vi "global.vi"() -> ()   [LabVIEW 2015]
panel:
  out "stop":bool
  out "crashed":bool
  out "FG Data":T1
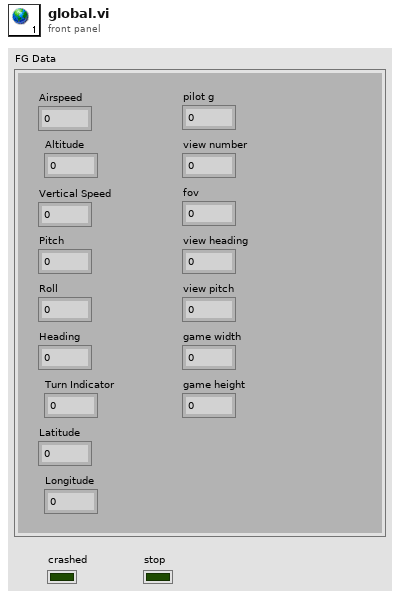
[diagram p1: front panel]
types:
  T1 = cluster{"Airspeed":dbl, "Altitude":dbl, "Vertical Speed":dbl, "Pitch":dbl, "Roll":dbl, "Heading":dbl, "Turn Indicator":dbl, "Latitude":dbl, "Longitude":dbl, "pilot g":dbl, "view number":i16, "fov":dbl, "view heading":dbl, "view pitch":dbl, "game width":i16, "game height":i16}
diagram:
